vi "Configure Von Operation.vi"(8 "error in (no error)":errorcluster, 9 "Voff Voltage (0 V)":dbl min=0.0 max=500.0 step=0.01 format="%.2g", 10 "Von Voltage (0 V)":dbl min=0.0 max=500.0 step=0.01 format="%.2g", 11 "VISA resource name":refnum<visa-resource-name>) -> (0 "error out":errorcluster, 3 "VISA resource name out":refnum<visa-resource-name>)   [LabVIEW 2019, in "BK Precision 8500B Series.lvlib"]
doc: "Configures the Von operation, which control the voltage turn on and off state for the electronic load. \n\nNote: When the input voltage exceeds the Von voltage value, the electronic load’s input state turns on. When the voltage goes below the Voff Voltage value, the electronic load's input state turns off. \nThis function can protect a DUT when its voltage goes below a specified level."
uses:
  <instrlib>/BK Precision 8500B Series/BK Precision 8500B Series.lvlib
panel:
  # "V"
  # "V"
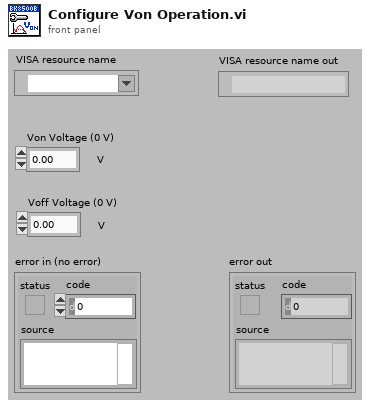
[diagram p1: front panel]
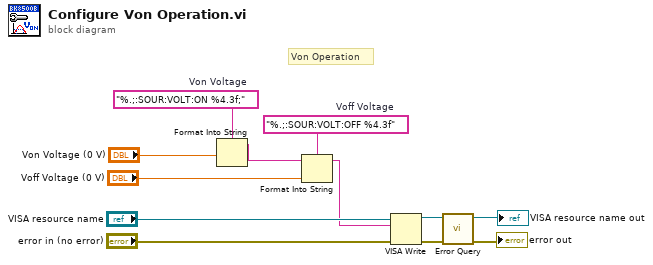
[diagram p0: block diagram]
diagram:
  w4 = "%.;:SOUR:VOLT:OFF %4.3f"  # Voff Voltage
  w8 = "%.;:SOUR:VOLT:ON %4.3f;"  # Von Voltage
  # "Von Operation"
  n1 = Format Into String(format string=w8, "Von Voltage (0 V)") -> (resulting string=w3:string)  [unwired: 2 in, 1 out]
  n2 = Format Into String(format string=w4, initial string=w3, "Voff Voltage (0 V)") -> (resulting string=w2:string)  [unwired: 1 in, 1 out]
  n3 = VISA Write(VISA resource name="VISA resource name", write buffer=w2, error in (no error)="error in (no error)") -> (VISA resource name out=w11:refnum<visa-resource-name>, error out=w12:errorcluster)  [unwired: 1 out]
  n4 = call <instrlib>:"Error Query.vi"("error in (no error)"=w12, "VISA resource name"=w11) -> ("error out"=→"error out":errorcluster, "VISA resource name out"=→"VISA resource name out":refnum<visa-resource-name>)  [unwired: 6 in, 2 out]
